vi "Get Child Libraries.vi"(8 "error in (no error)":errorcluster {"code" format="Error %.0f"}, 11 "Library Documentation In":refnum<class "Library Documentation.lvclass">) -> (0 "error out":errorcluster {"code" format="Error %.0f"}, 2 "Child Libraries":T1[](array[typedef]), 3 "Library Documentation Out":refnum<class "Library Documentation.lvclass">)   [LabVIEW 2023, in "VIDoc Parsing.lvlib" / "Library Documentation.lvclass"]
uses:
  Library Documentation.lvclass
  Child Libraries Cluster.ctl
  Library Documentation.lvclass/Library Documentation.ctl
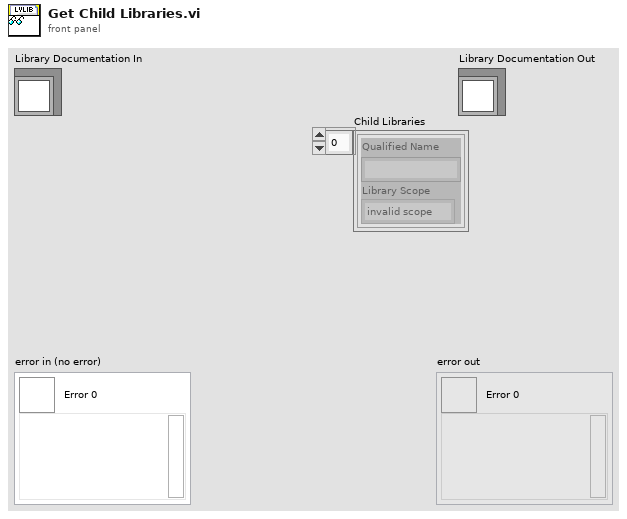
[diagram p1: front panel]
types:
  T1 = typedef "VIDoc Parsing.lvlib/Library Documentation.lvclass/Child Libraries Cluster.ctl" = cluster{"Qualified Name":string, "Library Scope":enum32{"invalid scope", "public", "private", "protected", "community"}}
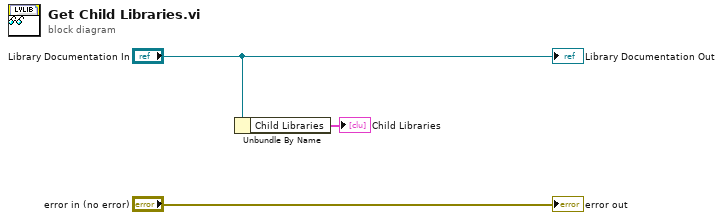
[diagram p0: block diagram]
diagram:
  n1 = Unbundle By Name("Library Documentation In") -> ("Child Libraries"=→"Child Libraries":T1[])
  "error out" <- "error in (no error)"
  "Library Documentation Out" <- "Library Documentation In"
